vi "Lightfield.vi"() -> ()   [LabVIEW 2018]
uses:
  C:/Program Files/Princeton Instruments/LightField/PrincetonInstruments.LightFieldAddInSupportServices.dll
  Program Files/Princeton Instruments/LightField/PrincetonInstruments.LightFieldAddInSupportServices.dll
  ProgramData/Documents/Princeton Instruments/LightField/Add-in and Automation SDK/Samples/LabVIEW Automation/lightfield-automation-labview/LightField Automation.lvclass
panel:
  in  "Save raw Image":bool
  in  "Stop After this Acquisition":bool=TRUE
  out "New File":bool
  in  "Acuisition type":enum16{"Repetitive", "Sequential"}(ring)=enum."Sequential"
  out "Time":dbl=650.0
  out "acquiring data":bool
  in  "Acquire":bool
  in  "Capture":bool
  out "Gate End":dbl=5600.0
  in  "Gate Width":dbl=50.0 min=0.5 format="%#_13g"
  in  "# Frames":i32=100 min=1
  in  "Gate Start":dbl=650.0 min=1.0 format="%#_13g"
  in  "File":enum32{"File"}(tab)
  in  "Filename":string="PL_10Hz_Rb_3"
  out "file path":path=path "E:/Alkali metals/Excimer/PL/2018-03-21/PL_10Hz_Rb_3.tdms"
  in  "base path":path=path "E:/Alkali metals/Excimer/PL"
  out "Lightfieldpath":path=path "E:/Alkali metals/Excimer/PL/2018-03-21/LightfieldRaw"
  out "File Size":i64=50126
  in  "Reset capture number":bool
  out "Capture number":i32=3
  in  "Frame":i32
  in  "Tab Control":enum32{"Imaging", "Spectral"}(tab)=enum."Spectral"
  out "Power vs Gate Delay":cluster{dbl[], dbl[]}(graph)={[740.0, 750.0, 760.0, 770.0, 780.0, 790.0, 800.0, 810.0, 820.0, 830.0, 840.0, 850.0, 860.0], [9735.629577636719, 9727.297424316406, 9722.783203125, 9721.853454589844, 9723.992553710938, 9728.69384765625, 9735.276550292969, 9743.003845214844, 9751.08984375, 9758.719848632812, 9764.941833496094, 9768.833984375, 9769.806823730469]}
  out "Gate delay of peak vs time":dbl[](graph)=[860.0]
  out "Capture ROI 1, Frame 2":dbl[][](graph)
  in  "BeamProfilelExperimentName":string="Vaportube_camera_sequential"
  out "Integrated peak vs gate delay":cluster{dbl[], dbl[]}(graph)={[650.0, 700.0, 750.0, 800.0, 850.0, 900.0, 950.0, 1000.0, 1050.0, 1100.0, 1150.0, 1200.0, 1250.0, 1300.0, 1350.0, 1400.0, 1450.0, 1500.0, 1550.0, 1600.0, 1650.0, 1700.0, 1750.0, 1800.0, 1850.0, 1900.0], [368.725, 81.825, 163.675, 339.125, 243.575, 82.55, -16.925, 60.325, 161.775, 63.55, 6.325, 69.075, -40.375, 4.375, 94.0, -26.325, -36.025, -132.65, -113.375, 22.05, -70.375, 7.35, -80.125, 60.75, -80.725, -112.075]}
  in  "Integration Center WL":dbl=770.0 format="%#_13g"
  in  "WL width":dbl=5.0 format="%#_13g"
  out "Spectrum":T1(graph)
  in  "Center Wavelength":dbl=790.0
  in  "SpectralExperimentName":string="Vaportube_PL_sequential"
  in  "Camera Setup":enum16{"Imaging", "Spectral"}(ring)=enum."Spectral"
  in  "Remove first page?":bool
  out "TDMS error":errorcluster
  out "TDMS file":refnum<k34>
  in  "stop":bool
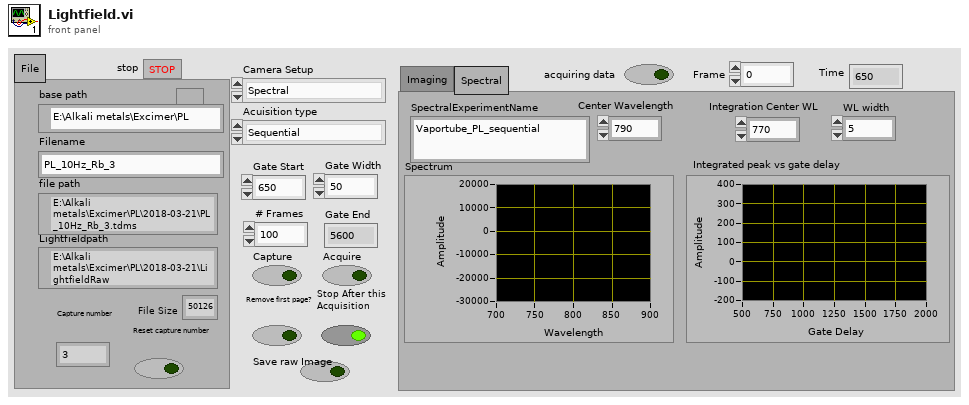
[diagram p1: front panel]
types:
  T1 = cluster{"ColumnCalibration":dbl[], "Image":dbl[]}
  T2 = cluster{"Image":dbl[][][], "Frame Size":cluster{"F":i32, "Y":i32, "X":i32}}[]
  T3 = cluster{"Image":dbl[][][], "Frame Size":cluster{"F":i32, "Y":i32, "X":i32}}
  T4 = cluster{"Gate Delay Array":dbl[], "Integrated emission vs gate delay":dbl[]}
  T5 = cluster{"Gate Delay Array":dbl[], "Avg Power each frame":dbl[]}
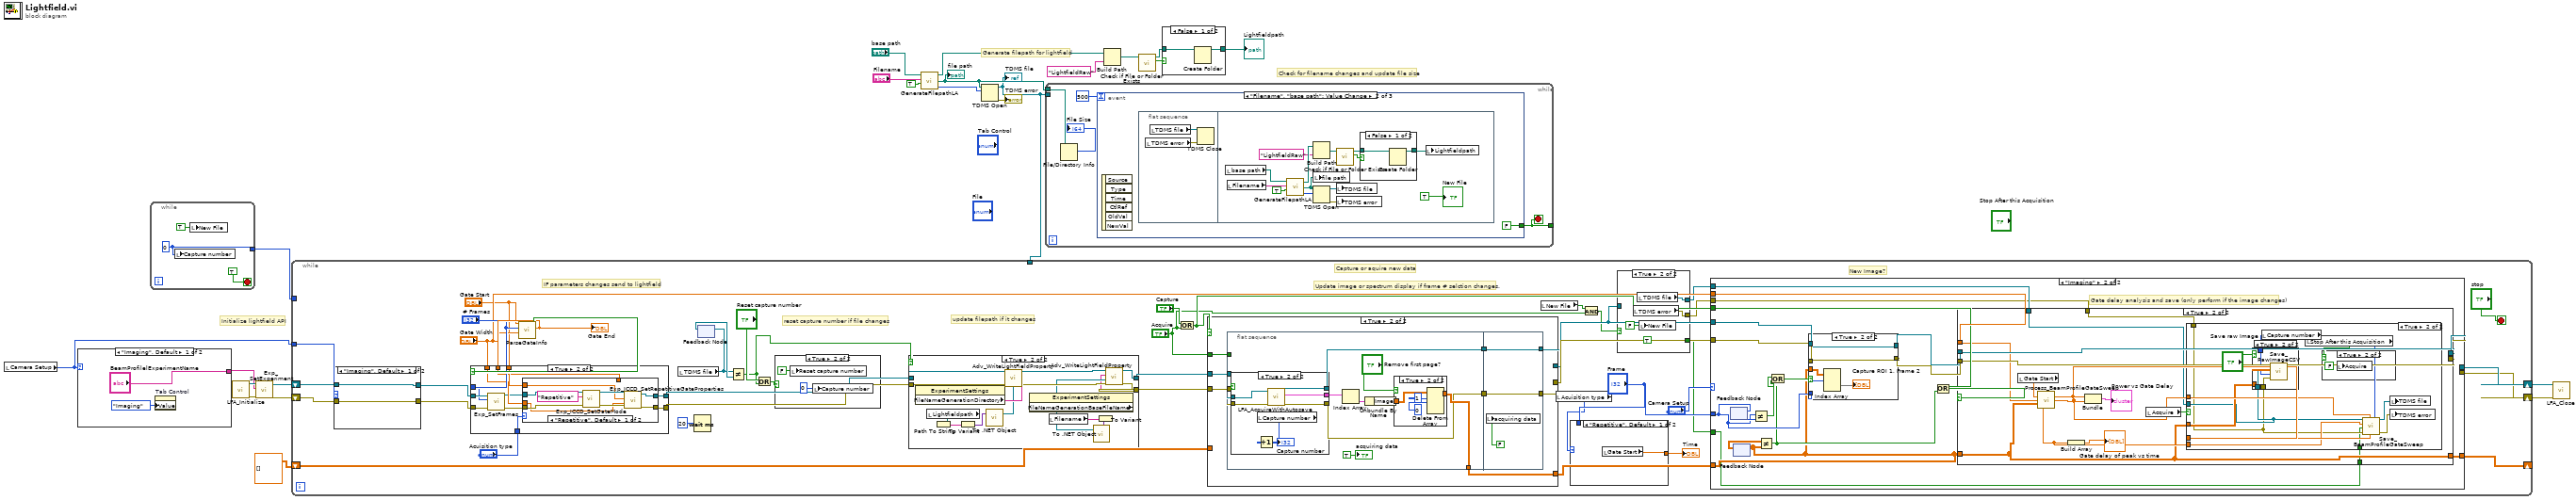
[diagram p0: block diagram]
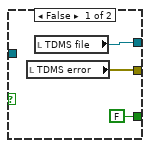
[diagram p2: hidden frame]
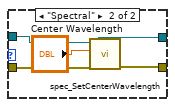
[diagram p3: hidden frame]
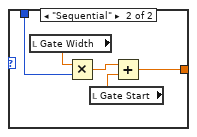
[diagram p4: hidden frame]
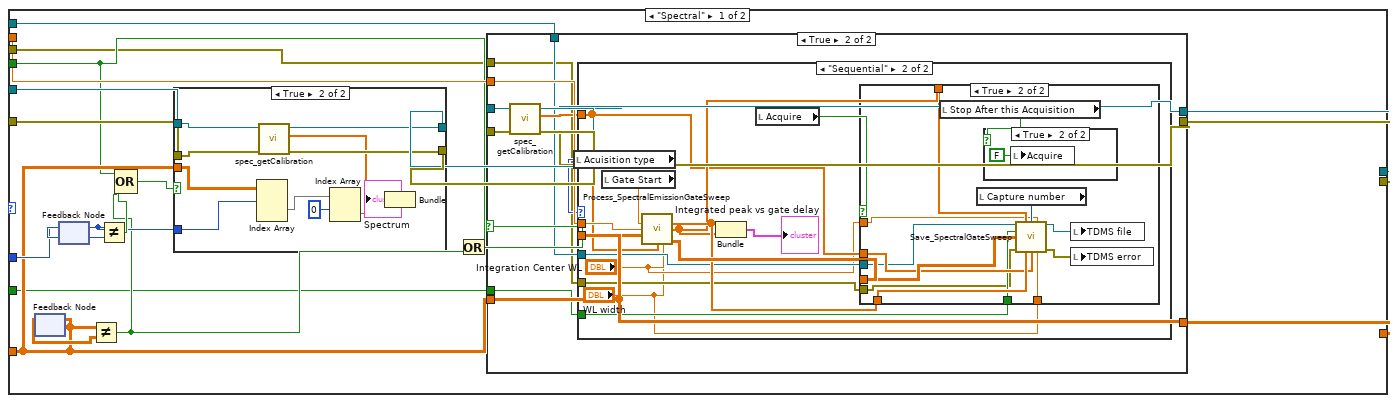
[diagram p5: hidden frame]
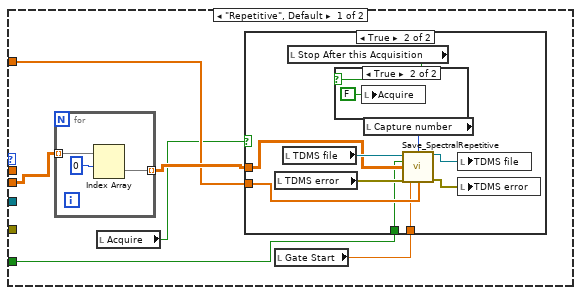
[diagram p8: hidden frame]
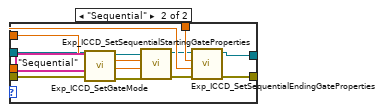
[diagram p19: hidden frame]
diagram:
  # "Check for filename changes and update file size"
  # "Initialize lightfield API"
  # "Generate filepath for lightfield"
  n1 = local read "Camera Setup"() -> (w1:enum16{"Imaging", "Spectral"})
  n2 = case shown="\"Imaging\", Default" w1 {
    tunnel: ["BeamProfilelExperimentName" "SpectralExperimentName"] -> w13
    frame "Imaging", Default {
      n3 = property on="Tab Control" class="TabCtl (strict)"("Value"=enum32{"Imaging", "Spectral"}."Imaging" ("Tab Control")) -> ()  [unwired: 2 in, 2 out]
    }
    frame "Spectral" {
      n4 = property on="Tab Control" class="TabCtl (strict)"("Value"=enum32{"Imaging", "Spectral"}."Spectral" ("Tab Control")) -> ()  [unwired: 2 in, 2 out]
    }
  }
  n5 = while {
    tunnel: [w29] -> w7
    stop <- TRUE stop-if-true
    w29 = 0 ("Capture number")
    n6 = local write "Capture number"(w29) -> ()
    n7 = local write "New File"(TRUE ("New File")) -> ()
  }
  n8 = call "LFA_Initialize.vi"() -> ("error out"=w14:errorcluster, "LightField Automation out"=w15:refnum<class "LightField Automation.lvclass">)  [unwired: 10 in]
  n9 = call "Exp_SetExperiment.vi"("error in (no error)"=w14, "ExperimentName"=w13, "LightField Automation in"=w15) -> ("error out"=w12:errorcluster, "LightField Automation out"=w11:refnum<class "LightField Automation.lvclass">)  [unwired: 7 in]
  n10 = call "GenerateFilepathLA.vi"("Auto Date folder"=TRUE, "Filename"="Filename", "base path"="base path") -> ("Numeric"=w19:i32, "file path"=w18:path, "Folder Path"=w17:path)  [unwired: 1 in]
  "file path" <- w18
  n11 = TDMS Open(10:w19, 11:w18) -> (0:→"TDMS error":errorcluster, 3:w2:refnum<k34>)  [unwired: 5 in]
  "TDMS file" <- w2
  n12 = while {
    shift-right: [w70] -> w9
    shift-left: w11 -> [w42]
    shift-right: [w69] -> w10
    shift-left: w12 -> [w41]
    shift-right: [w49] -> _
    shift-left: dbl[][][] [] ("Image") -> [w52]
    tunnel: w7 -> [_]
    tunnel: w2 -> [_]
    tunnel: w1 -> [w38]
    stop <- "stop" stop-if-true
    # "New Image?"
    # "Update image or spectrum display if frame # selction changes."
    # "Capture or aquire new data"
    # "reset capture number if file changes"
    # "update filepath if it changes"
    # "IF parameters changes send to lightfield"
    n13 = case shown="\"Imaging\", Default" w38 {
      tunnel: [w80 w84] -> w40
      tunnel: w42 -> [w80 w85]
      tunnel: [w79 w82] -> w39
      tunnel: w41 -> [w79 w83]
      frame "Imaging", Default {
      }
      frame "Spectral" {
        n14 = call "spec_SetCenterWavelength.vi"("error in (no error)"=w83, "Center Wavelength"="Center Wavelength", "LightField Automation in"=w85) -> ("error out"=w82:errorcluster, "LightField Automation out"=w84:refnum<class "LightField Automation.lvclass">)  [unwired: 7 in]
      }
    }
    n15 = call "ParseGateInfo.vi"("Gate Width"="Gate Width", "# Frames"="# Frames", "Gate Start"="Gate Start") -> ("Numeric"=w66:dbl, "Boolean"=w68:bool)  [unwired: 7 in]
    "Gate End" <- w66
    n16 = case shown="True" w68 {
      tunnel: w40 -> [w249 w255]
      tunnel: w39 -> [w248 w254]
      tunnel: "Gate Start" -> [_ w260]
      tunnel: [w249 w258] -> w62
      tunnel: [w248 w257] -> w61
      tunnel: w66 -> [_ w259]
      tunnel: "Gate Width" -> [_ w256]
      tunnel: "# Frames" -> [_ w251]
      tunnel: "Acuisition type" -> [_ w250]
      frame False {
      }
      frame True {
        n17 = call "Exp_SetFrames.vi"("error in (no error)"=w254, "Number of Frames"=w251, "LightField Automation in"=w255) -> ("error out"=w253:errorcluster, "LightField Automation out"=w252:refnum<class "LightField Automation.lvclass">)  [unwired: 7 in]
        n18 = case shown="\"Repetitive\", Default" w250 {
          tunnel: w260 -> [w262 w281]
          tunnel: w259 -> [_ w280]
          tunnel: [w266 w279] -> w258
          tunnel: [w264 w278] -> w257
          tunnel: w256 -> [w261 w277]
          tunnel: w253 -> [w268 w272]
          tunnel: w252 -> [w269 w274]
          frame "Repetitive", Default {
            n19 = call "Exp_ICCD_SetGateMode.vi"("error in (no error)"=w268, "Gate Mode"="Repetitive", "LightField Automation in"=w269) -> ("error out"=w265:errorcluster, "LightField Automation out"=w267:refnum<class "LightField Automation.lvclass">)  [unwired: 7 in]
            n20 = call "Exp_ICCD_SetRepetitiveGateProperties.vi"("error in (no error)"=w265, "Repetitive Gate Width (ns)"=w261, "Repetitive Gate Delay (ns)"=w262, "LightField Automation in"=w267) -> ("error out"=w264:errorcluster, "LightField Automation out"=w266:refnum<class "LightField Automation.lvclass">)  [unwired: 6 in]
          }
          frame "Sequential" {
            n21 = call "Exp_ICCD_SetGateMode.vi"("error in (no error)"=w272, "Gate Mode"="Sequential", "LightField Automation in"=w274) -> ("error out"=w271:errorcluster, "LightField Automation out"=w273:refnum<class "LightField Automation.lvclass">)  [unwired: 7 in]
            n22 = call "Exp_ICCD_SetSequentialStartingGateProperties.vi"("error in (no error)"=w271, "Sequential Starting Gate Width (ns)"=w277, "Sequential Starting Gate Delay (ns)"=w281, "LightField Automation in"=w273) -> ("error out"=w275:errorcluster, "LightField Automation out"=w276:refnum<class "LightField Automation.lvclass">)  [unwired: 6 in]
            n23 = call "Exp_ICCD_SetSequentialEndingGateProperties.vi"("error in (no error)"=w275, "Sequential Ending Gate Width (ns)"=w277, "Sequential Ending Gate Delay (ns)"=w280, "LightField Automation in"=w276) -> ("error out"=w278:errorcluster, "LightField Automation out"=w279:refnum<class "LightField Automation.lvclass">)  [unwired: 6 in]
          }
        }
      }
    }
    n24 = local read "TDMS file"() -> (w59:refnum<k34>)
    n25 = Wait (ms)(milliseconds to wait=u32 20) -> ()  [unwired: 1 out]
    n26 = feedback #1() -> (w60:refnum<k34>)  [unwired: 1 in]
    n27 = feedback-in #1(w59) -> ()
    n28 = Not Equal?(x=w59, y=w60) -> (x != y?=w56:bool)
    n29 = Or(x="Reset capture number", y=w56) -> (x .or. y?=w55:bool)
    n30 = case shown="True" w55 {
      frame False {
      }
      frame True {
        n31 = local write "Reset capture number"(FALSE ("Reset")) -> ()
        n32 = local write "Capture number"(0 ("Capture number")) -> ()
      }
    }
    n33 = case shown="True" w56 {
      tunnel: w62 -> [w327 w342]
      tunnel: w61 -> [w326 w341]
      tunnel: [w327 w333] -> w54
      tunnel: [w326 w332] -> w53
      frame False {
      }
      frame True {
        n34 = property class="ExperimentSettings"() -> ("FileNameGenerationDirectory"=w338:string)  [unwired: 2 in, 2 out]
        n35 = local read "Lightfieldpath"() -> (w336:path)
        n36 = Path To String(path=w336) -> (string=w340:string)
        n37 = To Variant(anything=w340) -> (Variant=w339:variant)
        n38 = call <vilib>:"To .NET Object.vi"("anything"=w339) -> (".NET object"=w337:refnum<k24>)  [unwired: 1 in, 1 out]
        n39 = call "Adv_WriteLightFieldProperty.vi"("error in (no error)"=w341, "value"=w337, "setting"=w338, "LightField Automation in"=w342) -> ("error out"=w330:errorcluster, "LightField Automation out"=w331:refnum<class "LightField Automation.lvclass">)  [unwired: 6 in]
        n40 = property class="ExperimentSettings"() -> ("FileNameGenerationBaseFileName"=w328:string)  [unwired: 2 in, 2 out]
        n41 = local read "Filename"() -> (w334:string)
        n42 = To Variant(anything=w334) -> (Variant=w335:variant)
        n43 = call <vilib>:"To .NET Object.vi"("anything"=w335) -> (".NET object"=w329:refnum<k24>)  [unwired: 1 in, 1 out]
        n44 = call "Adv_WriteLightFieldProperty.vi"("error in (no error)"=w330, "value"=w329, "setting"=w328, "LightField Automation in"=w331) -> ("error out"=w332:errorcluster, "LightField Automation out"=w333:refnum<class "LightField Automation.lvclass">)  [unwired: 6 in]
      }
    }
    n45 = Or(x="Capture", y="Acquire") -> (x .or. y?=w48:bool)
    n46 = case shown="True" w48 {
      tunnel: "Acquire" -> [_ w294]
      tunnel: w54 -> [w286 w293]
      tunnel: w53 -> [w285 w292]
      tunnel: [w284 w291] -> w50
      tunnel: [w286 w290] -> w34
      tunnel: [w285 w289] -> w51
      tunnel: w52 -> [w284 _]
      frame False {
      }
      frame True {
        n47 = flat-sequence {
          tunnel: [w300] -> w291
          tunnel: [w297] -> w288
          tunnel: [w296] -> w287
          tunnel: w294 -> [w305]
          tunnel: w293 -> [w304]
          tunnel: w292 -> [w303]
          tunnel: [w324] -> w289
          tunnel: [w325] -> w290
          tunnel: w288 -> [w325]
          tunnel: w287 -> [w324]
          frame #0 {
            n48 = case shown="True" w305 {
              tunnel: [w315 w319] -> w296
              tunnel: [w314 w321] -> w297
              tunnel: [w313 w318] -> w301
              tunnel: w304 -> [w312 w322]
              tunnel: w303 -> [w311 w320]
              frame False {
                n49 = call "LFA_Capture.vi"("error in (no error)"=w311, "LightField Automation in"=w312) -> ("error out"=w315:errorcluster, "Data"=w313:T2, "LightField Automation out"=w314:refnum<class "LightField Automation.lvclass">)  [unwired: 7 in]
              }
              frame True {
                n50 = local read "Capture number"() -> (w316:i32)
                n51 = Increment(x=w316) -> (x+1=→"Capture number":i32)
                n52 = call "LFA_AcquireWithAutosave.vi"("error in (no error)"=w320, "LightField Automation in"=w322) -> ("error out"=w319:errorcluster, "Data"=w318:T2, "LightField Automation out"=w321:refnum<class "LightField Automation.lvclass">)  [unwired: 7 in]
              }
            }
            n53 = Index Array(array=w301) -> (element=w302:T3)  [unwired: 1 in]
            n54 = Unbundle By Name(w302) -> ("Image"=w299:dbl[][][])
            n55 = case shown="True" "Remove first page?" {
              tunnel: [w306 w310] -> w300
              tunnel: w299 -> [w306 w309]
              frame False {
              }
              frame True {
                n56 = Delete From Array(array=w309, length=1, index (dim 0)=0 ("index (page)")) -> (array with subset deleted=w310:dbl[][][])  [unwired: 2 in, 1 out]
              }
            }
            "acquiring data" <- TRUE ("aquiring data")
          }
          frame #1 {
            n57 = local write "acquiring data"(FALSE ("aquiring data")) -> ()
          }
        }
      }
    }
    n58 = local read "New File"() -> (w33:bool)
    n59 = local read "Acuisition type"() -> (w43:enum16{"Repetitive", "Sequential"})
    n60 = case shown="\"Repetitive\", Default" w43 {
      tunnel: [w86 w91] -> w46
      tunnel: "Frame" -> [_ w87]
      frame "Repetitive", Default {
        n61 = local read "Gate Start"() -> (w86:dbl)
      }
      frame "Sequential" {
        n62 = local read "Gate Width"() -> (w88:dbl)
        n63 = Multiply(x=w88, y=w87) -> (x*y=w89:dbl)
        n64 = local read "Gate Start"() -> (w90:dbl)
        n65 = Add(x=w89, y=w90) -> (x+y=w91:dbl)
      }
    }
    "Time" <- w46
    n66 = And(x=w33, y="Acquire") -> (x .and. y?=w31:bool)
    n67 = case shown="True" w31 {
      tunnel: [FALSE ("New File") TRUE ("New File")] -> w37
      tunnel: [w73 w76] -> w36
      tunnel: [w72 w75] -> w35
      tunnel: w34 -> [_ _]
      frame False {
        n68 = local read "TDMS error"() -> (w72:errorcluster)
        n69 = local read "TDMS file"() -> (w73:refnum<k34>)
      }
      frame True {
        n70 = local read "TDMS error"() -> (w75:errorcluster)
        n71 = local read "TDMS file"() -> (w76:refnum<k34>)
        n72 = local write "New File"(FALSE ("New File")) -> ()
      }
    }
    n73 = case shown="\"Imaging\"" "Camera Setup" {
      tunnel: [w111 w206] -> w70
      tunnel: [w110 w205] -> w69
      tunnel: "Gate Width" -> [w109 w204]
      tunnel: "Frame" -> [w99 w194]
      tunnel: w34 -> [w107 w202]
      tunnel: w51 -> [w106 w201]
      tunnel: w50 -> [w97 w190]
      tunnel: [w100 w195] -> w49
      tunnel: w48 -> [w95 w193]
      tunnel: w37 -> [w94 w187]
      tunnel: w36 -> [w93 w189]
      tunnel: w35 -> [w92 w188]
      frame "Spectral" {
        n74 = feedback #2() -> (w98:dbl[][][])  [unwired: 1 in]
        n75 = feedback-in #2(w97) -> ()
        n76 = feedback #3() -> (w108:i32)  [unwired: 1 in]
        n77 = feedback-in #3(w99) -> ()
        n78 = Not Equal?(x=w97, y=w98) -> (x != y?=w96:bool)
        n79 = Not Equal?(x=w99, y=w108) -> (x != y?=w101:bool)
        n80 = Compound Arithmetic op=OR(w95, w96, w101) -> (w102:bool)
        n81 = case shown="True" w102 {
          tunnel: w107 -> [w113 w120]
          tunnel: w106 -> [w112 w119]
          tunnel: [w112 w117] -> w105
          tunnel: [w113 w118] -> w104
          tunnel: w99 -> [_ w124]
          tunnel: w97 -> [_ w121]
          frame False {
          }
          frame True {
            n82 = Index Array(array=w121, index (dim 0)=w124) -> (element=w123:dbl[][])  [unwired: 2 in]
            n83 = call "spec_getCalibration.vi"("error in (no error)"=w119, "LightField Automation in"=w120) -> ("error out"=w117:errorcluster, "ColumnCalibration"=w115:dbl[], "LightField Automation out"=w118:refnum<class "LightField Automation.lvclass">)  [unwired: 7 in]
            n84 = Index Array(array=w123, index (row)=0) -> (element=w116:dbl[])  [unwired: 1 in]
            n85 = Bundle("ColumnCalibration"=w115, "Image"=w116) -> (→"Spectrum":T1)  [unwired: 1 in]
          }
        }
        n86 = Or(x=w95, y=w96) -> (x .or. y?=w103:bool)
        n87 = case shown="True" w103 {
          tunnel: [w127 w138] -> w111
          tunnel: [w126 w137] -> w110
          tunnel: w109 -> [_ w136]
          tunnel: w105 -> [w126 w135]
          tunnel: w104 -> [w127 w134]
          tunnel: w97 -> [w125 w133]
          tunnel: [w125 w133] -> w100
          tunnel: w94 -> [_ w130]
          tunnel: w93 -> [_ w129]
          tunnel: w92 -> [_ w128]
          frame False {
          }
          frame True {
            n88 = call "spec_getCalibration.vi"("error in (no error)"=w135, "LightField Automation in"=w134) -> ("error out"=w137:errorcluster, "ColumnCalibration"=w132:dbl[], "LightField Automation out"=w138:refnum<class "LightField Automation.lvclass">)  [unwired: 7 in]
            n89 = local read "Acuisition type"() -> (w131:enum16{"Repetitive", "Sequential"})
            n90 = case shown="\"Sequential\"" w131 {
              tunnel: w136 -> [_ w172]
              tunnel: w133 -> [w144 w171]
              tunnel: w132 -> [w141 w164]
              tunnel: w130 -> [w139 w163]
              tunnel: w129 -> [_ w162]
              tunnel: w128 -> [_ w161]
              frame "Repetitive", Default {
                n91 = for {
                  tunnel: w144 -> [w146] mode=indexing
                  tunnel: [w145] -> w143 mode=indexing
                  n92 = Index Array(array=w146, index (row)=0) -> (element=w145:dbl[])  [unwired: 1 in]
                }
                n93 = local read "Acquire"() -> (w140:bool)
                n94 = local read "Gate Start"() -> (w142:dbl)
                n95 = case shown="True" w140 {
                  tunnel: w141 -> [_ w152]
                  tunnel: w143 -> [_ w150]
                  tunnel: w142 -> [_ w151]
                  tunnel: w139 -> [_ w149]
                  frame False {
                  }
                  frame True {
                    n96 = local read "TDMS error"() -> (w156:errorcluster)
                    n97 = local read "TDMS file"() -> (w157:refnum<k34>)
                    n98 = local read "Stop After this Acquisition"() -> (w148:bool)
                    n99 = case shown="True" w148 {
                      frame False {
                      }
                      frame True {
                        n100 = local write "Acquire"(FALSE ("Acquire")) -> ()
                      }
                    }
                    n101 = local read "Capture number"() -> (w153:i32)
                    n102 = call "Save_SpectralRepetitive.vi"("Refnum in"=w157, "Capture number"=w153, "New File"=w149, "Image"=w150, "error in (no error)"=w156, "Gate Delay"=w151, "Wavelength Array"=w152) -> ("Refnum out"=w155:refnum<k34>, "error out"=w154:errorcluster)  [unwired: 7 in]
                    n103 = local write "TDMS file"(w155) -> ()
                    n104 = local write "TDMS error"(w154) -> ()
                  }
                }
              }
              frame "Sequential" {
                n105 = local read "Gate Start"() -> (w168:dbl)
                n106 = call "Process_SpectralEmissionGateSweep.vi"("Center WL"="Integration Center WL", "Gate Start"=w168, "Gate Width"=w172, "Image"=w171, "ColumnCalibration"=w164, "WL width"="WL width") -> ("Gate Delay Array"=w166:dbl[], "Integrated emission vs gate delay"=w165:dbl[], "Spectra Array"=w169:dbl[][])  [unwired: 7 in]
                n107 = Bundle("Gate Delay Array"=w166, "Integrated emission vs gate delay"=w165) -> (→"Integrated peak vs gate delay":T4)  [unwired: 1 in]
                n108 = local read "Acquire"() -> (w167:bool)
                n109 = case shown="True" w167 {
                  tunnel: w169 -> [_ w182]
                  tunnel: w166 -> [_ w181]
                  tunnel: w165 -> [_ w179]
                  tunnel: w164 -> [_ w180]
                  tunnel: w163 -> [_ w178]
                  tunnel: w162 -> [_ w176]
                  tunnel: w161 -> [_ w175]
                  tunnel: "Integration Center WL" -> [_ w174]
                  tunnel: "WL width" -> [_ w173]
                  frame False {
                  }
                  frame True {
                    n110 = local read "Stop After this Acquisition"() -> (w177:bool)
                    n111 = local read "Capture number"() -> (w183:i32)
                    n112 = case shown="True" w177 {
                      frame False {
                      }
                      frame True {
                        n113 = local write "Acquire"(FALSE ("Acquire")) -> ()
                      }
                    }
                    n114 = call "Save_SpectralGateSweep.vi"("Refnum in"=w176, "Integrated Emission"=w179, "Capture number"=w183, "Integration Center WL"=w174, "New file"=w178, "Image"=w182, "error in (no error)"=w175, "Gate Delay array"=w181, "Wavelength Array"=w180, "WL width"=w173) -> ("Refnum out"=w185:refnum<k34>, "error out"=w184:errorcluster)  [unwired: 4 in]
                    n115 = local write "TDMS file"(w185) -> ()
                    n116 = local write "TDMS error"(w184) -> ()
                  }
                }
              }
            }
          }
        }
      }
      frame "Imaging" {
        # "Gate delay analysis and save (only perform if the image changes)"
        n117 = feedback #4() -> (w203:i32)  [unwired: 1 in]
        n118 = feedback-in #4(w194) -> ()
        n119 = feedback #5() -> (w192:dbl[][][])  [unwired: 1 in]
        n120 = feedback-in #5(w190) -> ()
        n121 = Not Equal?(x=w194, y=w203) -> (x != y?=w196:bool)
        n122 = Not Equal?(x=w192, y=w190) -> (x != y?=w191:bool)
        n123 = Or(x=w191, y=w196) -> (x .or. y?=w197:bool)
        n124 = case shown="True" w197 {
          tunnel: w194 -> [_ w213]
          tunnel: w202 -> [w208 w211]
          tunnel: w201 -> [w207 w212]
          tunnel: [w207 w212] -> w200
          tunnel: [w208 w211] -> w199
          tunnel: w190 -> [_ w209]
          frame False {
          }
          frame True {
            n125 = Index Array(array=w209, index (dim 0)=w213) -> (element=→"Capture ROI 1, Frame 2":dbl[][])  [unwired: 2 in]
          }
        }
        n126 = Or(x=w193, y=w191) -> (x .or. y?=w198:bool)
        n127 = case shown="True" w198 {
          tunnel: [w216 w230] -> w206
          tunnel: [w215 w229] -> w205
          tunnel: w204 -> [_ w228]
          tunnel: w200 -> [w215 w229]
          tunnel: w199 -> [w216 w230]
          tunnel: w190 -> [w214 w220]
          tunnel: [w214 w220] -> w195
          tunnel: w189 -> [_ w219]
          tunnel: w188 -> [_ w218]
          tunnel: w187 -> [_ w217]
          frame False {
          }
          frame True {
            n128 = local read "Gate Start"() -> (w225:dbl)
            n129 = call "Process_BeamProfileGateSweep.vi"("Gate Start"=w225, "Gate Width"=w228, "Image"=w220) -> ("Gate Delay Array"=w224:dbl[], "Avg Power each frame"=w223:dbl[], "Gate Delay of peak intensity"=w222:dbl)  [unwired: 10 in]
            n130 = Build Array(w222) -> (→"Gate delay of peak vs time":dbl[])
            n131 = Bundle("Gate Delay Array"=w224, "Avg Power each frame"=w223) -> (→"Power vs Gate Delay":T5)  [unwired: 1 in]
            n132 = local read "Acquire"() -> (w221:bool)
            n133 = case shown="True" w221 {
              tunnel: w224 -> [_ w240]
              tunnel: w223 -> [_ w239]
              tunnel: w222 -> [_ w238]
              tunnel: w220 -> [_ w236]
              tunnel: w219 -> [_ w233]
              tunnel: w218 -> [_ w232]
              tunnel: w217 -> [_ w231]
              frame False {
              }
              frame True {
                n134 = local read "Capture number"() -> (w234:i32)
                n135 = case shown="True" "Save raw Image" {
                  tunnel: w236 -> [_ w246]
                  tunnel: w233 -> [_ w245]
                  tunnel: w232 -> [_ w244]
                  tunnel: w234 -> [_ w243]
                  frame False {
                  }
                  frame True {
                    n136 = call "Save_RawImageCSV.vi"("error in (no error)"=w244, "Capture number"=w243, "Image"=w246, "TDMS file"=w245) -> ()  [unwired: 1 out]
                  }
                }
                n137 = local read "Stop After this Acquisition"() -> (w237:bool)
                n138 = case shown="True" w237 {
                  frame False {
                  }
                  frame True {
                    n139 = local write "Acquire"(FALSE ("Acquire")) -> ()
                  }
                }
                n140 = call "Save_BeamProfileGateSweep.vi"("Capture Number"=w234, "Gate Delay Array"=w240, "Average power"=w239, "Error In"=w232, "New File?"=w231, "Gate Delay of peak intensity"=w238, "File In"=w233) -> ("error out"=w241:errorcluster, "File Out"=w242:refnum<k34>)  [unwired: 3 in]
                n141 = local write "TDMS file"(w242) -> ()
                n142 = local write "TDMS error"(w241) -> ()
              }
            }
          }
        }
      }
    }
  }
  n143 = while {
    tunnel: [w343] -> _
    tunnel: w18 -> [w344]
    tunnel: w2 -> [_]
    stop <- w343 stop-if-true
    n144 = File/Directory Info(path=w344) -> (size=→"File Size":i64)  [unwired: 1 in, 6 out]
    n145 = event shown="[1] \"Filename\", \"base path\": Value Change" {
      selector: _ -> [_ _ _]
      dyn-events: _ -> [_ _ _]
      timeout: 500 -> [_ _ _]
      tunnel: [FALSE ("NewVal") FALSE ("NewVal") w370] -> w343
      event Timeout {
        n146 = event-data() -> ()  [unwired: 1 in, 3 out]
      }
      event "Filename", "base path": Value Change {
        n147 = event-data() -> ()  [unwired: 1 in, 6 out]
        n148 = flat-sequence {
          frame #0 {
            n149 = local read "TDMS error"() -> (w350:errorcluster)
            n150 = local read "TDMS file"() -> (w349:refnum<k34>)
            n151 = TDMS Close(8:w350, 11:w349) -> ()  [unwired: 2 out]
          }
          frame #1 {
            n152 = local read "base path"() -> (w364:path)
            n153 = local read "Filename"() -> (w358:string)
            n154 = call "GenerateFilepathLA.vi"("Auto Date folder"=TRUE, "Filename"=w358, "base path"=w364) -> ("Numeric"=w361:i32, "file path"=w363:path, "Folder Path"=w357:path)  [unwired: 1 in]
            n155 = Build Path(base path=w357, name or relative path="LightfieldRaw") -> (appended path=w355:path)
            n156 = local write "file path"(w363) -> ()
            n157 = TDMS Open(10:w361, 11:w363) -> (0:w359:errorcluster, 3:w360:refnum<k34>)  [unwired: 5 in]
            n158 = call <vilib>:"Check if File or Folder Exists.vi"("path"=w355) -> ("file or folder exists?"=w354:bool, "dup path"=w353:path)  [unwired: 8 in, 1 out]
            n159 = local write "TDMS file"(w360) -> ()
            n160 = local write "TDMS error"(w359) -> ()
            n161 = case shown="False" w354 {
              tunnel: w353 -> [w366 w367]
              tunnel: [w365 w367] -> w352
              frame False {
                n162 = Create Folder(path (use dialog)=w366) -> (created path=w365:path)  [unwired: 2 in, 2 out]
              }
              frame True {
              }
            }
            n163 = local write "Lightfieldpath"(w352) -> ()
            "New File" <- TRUE
          }
        }
      }
      event "stop": Value Change {
        n164 = event-data() -> ("NewVal"=w370:bool)  [unwired: 1 in, 5 out]
        n165 = local read "TDMS error"() -> (w369:errorcluster)
        n166 = local read "TDMS file"() -> (w368:refnum<k34>)
        n167 = TDMS Close(8:w369, 11:w368) -> ()  [unwired: 2 out]
      }
    }
  }
  n168 = Build Path(base path=w17, name or relative path="LightfieldRaw") -> (appended path=w3:path)
  n169 = call <vilib>:"Check if File or Folder Exists.vi"("path"=w3) -> ("file or folder exists?"=w5:bool, "dup path"=w6:path)  [unwired: 8 in, 1 out]
  n170 = case shown="False" w5 {
    tunnel: w6 -> [w372 w373]
    tunnel: [w371 w373] -> w4
    frame False {
      n171 = Create Folder(path (use dialog)=w372) -> (created path=w371:path)  [unwired: 2 in, 2 out]
    }
    frame True {
    }
  }
  "Lightfieldpath" <- w4
  n172 = call "LFA_Close.vi"("error in (no error)"=w10, "LightField Automation in"=w9) -> ()  [unwired: 8 in, 2 out]
